vi "Process.vi"(8 "error in (no error)":errorcluster, 11 "Execution Profiler In":refnum<class "Execution Profiler.lvclass">) -> (0 "error out":errorcluster, 3 "Execution Profiler Out":refnum<class "Execution Profiler.lvclass">)   [LabVIEW 2020, in "Execution Profiler.lvclass"]
uses:
  Execution Profiler.lvclass
  C:/git/astemes-lunit/source/Application Framework/Process Classes/Process/Process.lvclass
  User Interface/Process/Process.lvclass/Process.ctl
  <vilib>/Utility/error.llb/Error Cluster From Error Code.vi
  <vilib>/ErrorRing/Error Ring.xnode
  Execution Profiler.lvclass/Execution Profiler.ctl
  User Interface/Process/Process.lvclass
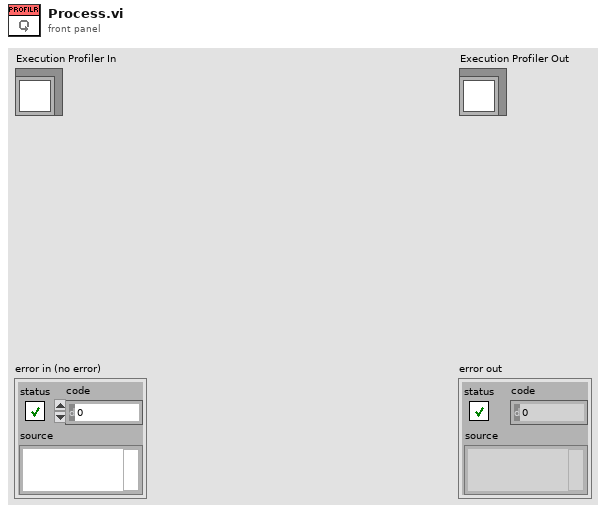
[diagram p1: front panel]
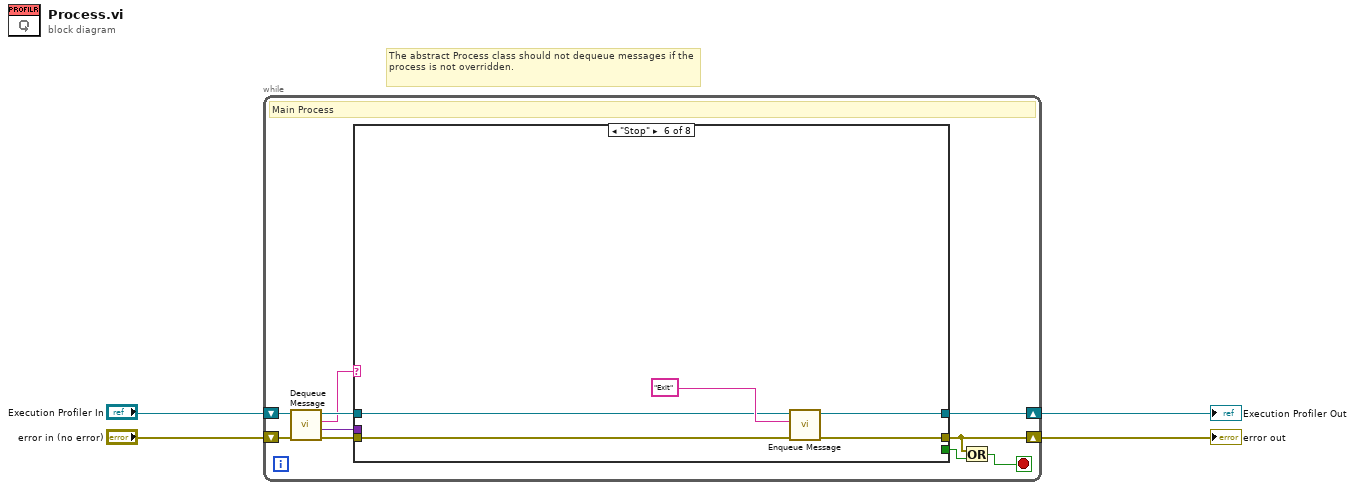
[diagram p0: block diagram]
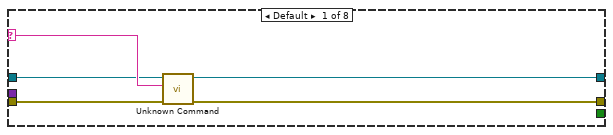
[diagram p2: hidden frame]
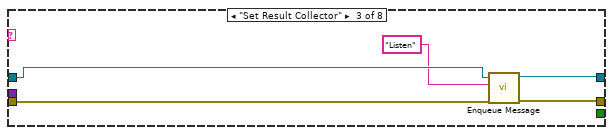
[diagram p4: hidden frame]
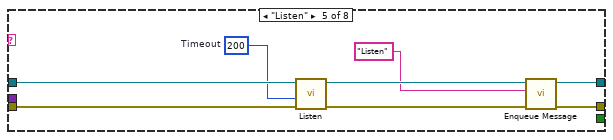
[diagram p6: hidden frame]
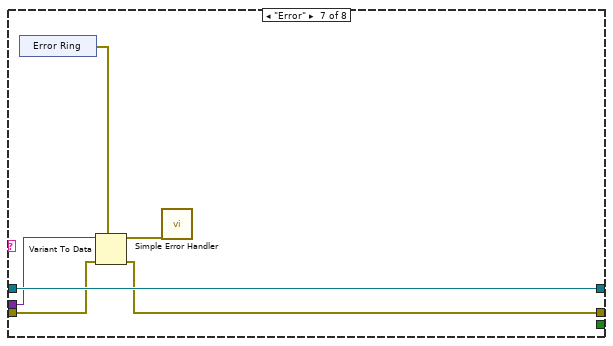
[diagram p7: hidden frame]
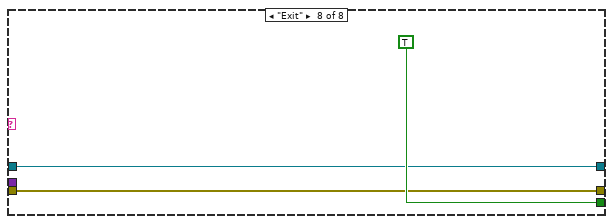
[diagram p8: hidden frame]
diagram:
  # "The abstract Process class should not dequeue messages if the process is not overridden."
  n1 = while {
    shift-right: [w6] -> w4
    shift-left: "error in (no error)" -> [w13]
    shift-right: [w5] -> w3
    shift-left: "Execution Profiler In" -> [w14]
    stop <- w7 stop-if-true
    # "Main Process"
    n2 = call "Dequeue Message.vi"("error in (no error)"=w13, "Process In"=w14) -> ("error out"=w12:errorcluster, "Message Data"=w9:variant, "Message"=w10:string, "Process Out"=w11:refnum<class "Execution Profiler.lvclass">)  [unwired: 6 in]
    n3 = case shown="\"Stop\"" w10 {
      selector: w10 -> [w19 _ _ _ _ _ _ _]
      tunnel: [w16 w21 w22 w28 w35 w39 w43 w49] -> w6
      tunnel: w12 -> [w15 w21 w26 w28 w33 w40 w46 w49]
      tunnel: [w18 w20 w23 w27 w36 w38 w47 w50] -> w5
      tunnel: w11 -> [w17 w20 w25 w27 w34 w37 w47 w50]
      tunnel: w9 -> [_ _ _ _ _ _ w45 _]
      tunnel: [_ _ _ _ _ _ _ TRUE] -> w8
      frame Default {
        n4 = call "Unknown Command.vi"("error in (no error)"=w15, "String"=w19, "Process In"=w17) -> ("error out"=w16:errorcluster, "Process Out"=w18:refnum<class "Execution Profiler.lvclass">)  [unwired: 7 in]
      }
      frame "Init" {
      }
      frame "Set Result Collector" {
        n5 = call "Enqueue Message.vi"("error in (no error)"=w26, "Message"="Listen", "Process In"=w25) -> ("error out"=w22:errorcluster, "Process Out"=w23:refnum<class "Execution Profiler.lvclass">)  [unwired: 7 in]
      }
      frame "Set Test Finder" {
      }
      frame "Listen" {
        w30 = 200  # Timeout
        n6 = call "Listen.vi"("error in (no error)"=w33, "Timeout"=w30, "Execution Profiler In"=w34) -> ("error out"=w31:errorcluster, "Execution Profiler Out"=w32:refnum<class "Execution Profiler.lvclass">)  [unwired: 7 in]
        n7 = call "Enqueue Message.vi"("error in (no error)"=w31, "Message"="Listen", "Process In"=w32) -> ("error out"=w35:errorcluster, "Process Out"=w36:refnum<class "Execution Profiler.lvclass">)  [unwired: 7 in]
      }
      frame "Stop" {
        n8 = call "Enqueue Message.vi"("error in (no error)"=w40, "Message"="Exit", "Process In"=w37) -> ("error out"=w39:errorcluster, "Process Out"=w38:refnum<class "Execution Profiler.lvclass">)  [unwired: 7 in]
      }
      frame "Error" {
        n9 = xnode "Error Ring"() -> ("error out"=w44:errorcluster)
        n10 = Variant To Data(error in=w46, type=w44, Variant=w45) -> (data=w42:errorcluster, error out=w43:errorcluster)
        n11 = call <vilib>:"Simple Error Handler.vi"("error in (no error)"=w42) -> ()  [unwired: 4 in, 5 out]
      }
      frame "Exit" {
      }
    }
    n12 = Or(x=w6, y=w8) -> (x .or. y?=w7:bool)
  }
  "error out" <- w4
  "Execution Profiler Out" <- w3
